vi "Ctor.vi"(8 "error in (no error)":errorcluster, 11 "Element Base in":refnum<class "Element Base.lvclass">) -> (0 "error out":errorcluster, 3 "Element Base out":refnum<class "Element Base.lvclass">)   [LabVIEW 2020, in "Element Base.lvclass"]
uses:
  Element Base.lvclass
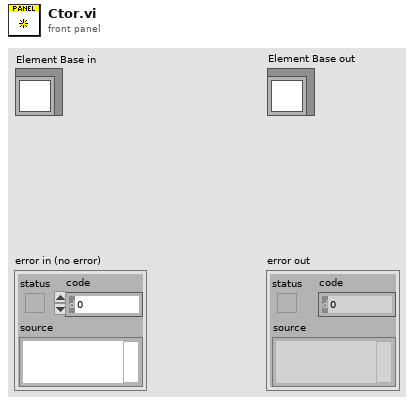
[diagram p1: front panel]
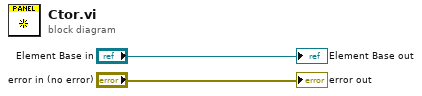
[diagram p0: block diagram]
diagram:
  "error out" <- "error in (no error)"
  "Element Base out" <- "Element Base in"
